vi "Initialize.vi"(8 "error in":errorcluster) -> (0 "error out":errorcluster, 3 "CutomOOB_Rx out":refnum<class "TemplateOOB_Rx.lvclass">)   [LabVIEW 2021, in "TemplateOOB_Rx.lvclass"]
uses:
  TemplateOOB_Rx.lvclass
  TemplateOOB_Rx.lvclass/TemplateOOB_Rx.ctl
  CIF-LVCore/src/CIFUtilities/CIFOutOfBand/CIFOutOfBand.lvclass
  Typedef/Payload.ctl
  D:/dev/CIF-LVCore/src/CIFUtilities/CIFOutOfBand/CIFOutOfBand.lvclass
  D:/dev/Plugins/Template/OOB/OOB_Rx/TemplateOOB_Rx.lvclass
  Typedef/Cyclic Data.ctl
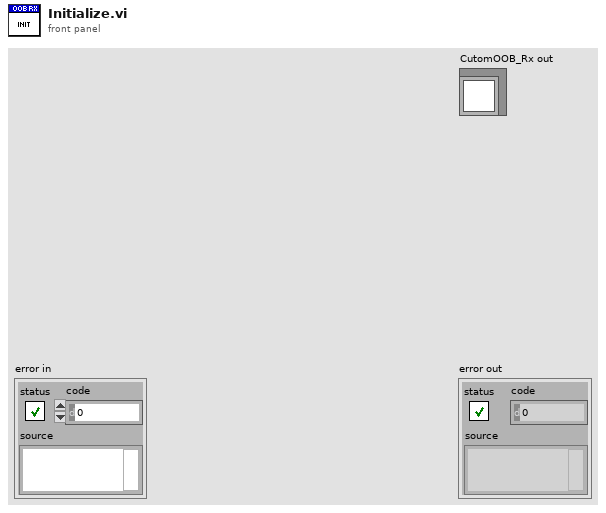
[diagram p1: front panel]
types:
  T1 = typedef "TemplateOOB_Rx.lvclass/Payload.ctl" = cluster{"Data":T2}
  T2 = typedef "TemplateOOB_Rx.lvclass/Cyclic Data.ctl" = cluster{"Numeric":i32}
  T3 = typedef "TemplateOOB_Rx.lvclass/Command Setting Control.ctl" = cluster{"Enum":T4, "U8":u8, " Payload":bool}
  T4 = typedef "TemplateOOB_Rx.lvclass/OOB Commands.ctl" = enum8{"Update Data"}
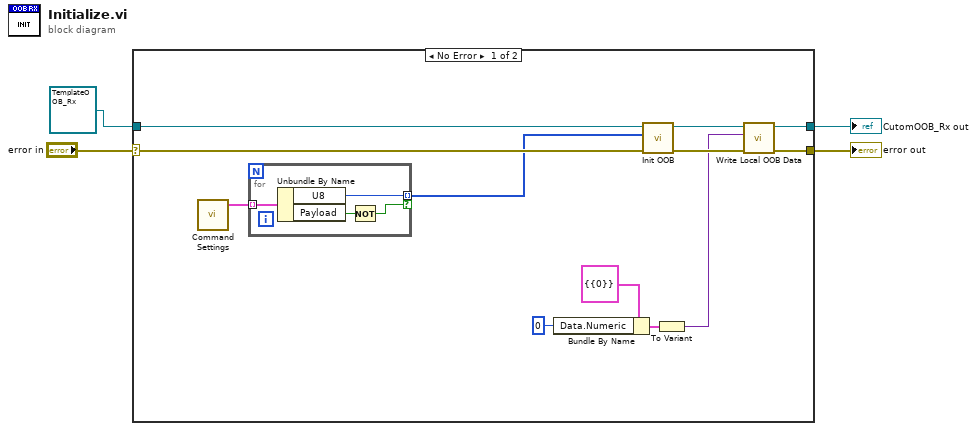
[diagram p0: block diagram]
diagram:
  n1 = case shown="No Error" "error in" {
    selector: "error in" -> [w16 w22]
    tunnel: [w10 w22] -> w3
    tunnel: [w11 w21] -> w2
    tunnel: refnum<class "TemplateOOB_Rx.lvclass"> refnum ("CifLvTemplateOutOfBand in") -> [w5 w21]
    frame No Error {
      n2 = call "Command Settings.vi"() -> ("Command Settings"=w15:T3[])  [unwired: 5 in]
      n3 = for {
        tunnel: w15 -> [w20] mode=indexing
        tunnel: [w19] -> w14 mode=indexing if=w17
        n4 = Unbundle By Name(w20) -> ("U8"=w19:u8, "Payload"=w18:bool)
        n5 = Not(x=w18) -> (.not. x?=w17:bool)
      }
      n6 = Bundle By Name(cluster=T1 {"Data"={"Numeric"=0}} ("Template Payload"), "Data.Numeric"=0) -> (w8:T1)
      n7 = call "Init OOB.vi"("error in (no error)"=w16, "Cases to Skip Payload"=w14, "OOB in"=w5) -> ("error out"=w13:errorcluster, "OOB out"=w12:refnum<class "TemplateOOB_Rx.lvclass">)  [unwired: 7 in]
      n8 = To Variant(anything=w8) -> (Variant=w7:variant)
      n9 = call "Write Local OOB Data.vi"("error in"=w13, "Local OOB Data"=w7, "OOB in"=w12) -> ("error out"=w10:errorcluster, "OOB out"=w11:refnum<class "TemplateOOB_Rx.lvclass">)  [unwired: 7 in]
    }
    frame Error {
    }
  }
  "error out" <- w3
  "CutomOOB_Rx out" <- w2
